vi "Sequence.Build.vi"(8 "error in (no error)":errorcluster, 11 "State Variables":T1={"Aliases.All"=[], "Aliases.Outputs"=[], "UI.Sequence#ofColumns"=0, "SysDef.Path"=path "", "UI.SequenceRef"=refnum, "UI.StepInformationRef"=refnum, "UI.AbortRef"=refnum, "UI.GraphRef"=refnum, "UI.ViewRef"=refnum, "UI.IterationsRef"=refnum, "UI.IterationInformationRef"=refnum, "INI.Settings"={"Build Location"=path "C:/Simple Sequence Editor/SequenceRepo", "LoggingLocation"=path ""}}) -> (0 "error out":errorcluster)   [LabVIEW 2013, in "Simple Sequence Tools - Editor.lvlib"]
uses:
  Simple Sequence Tools - Editor.lvlib
  Types/StateVariables.ctl
  Shared/Types/ChannelProperties.ctl
  Shared/Types/INI.Settings
  Shared/Simple Sequence Tools - Shared.lvlib
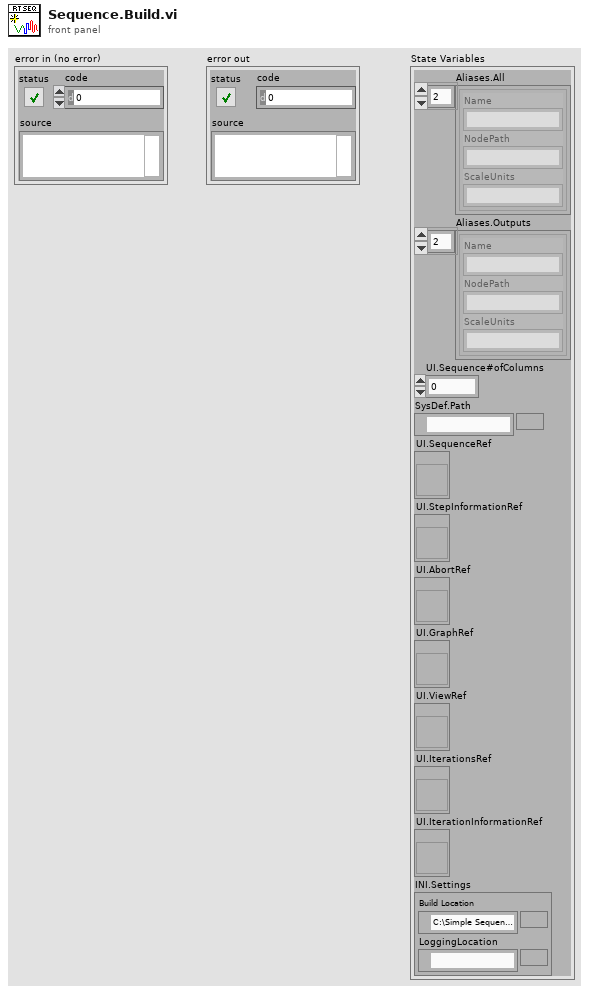
[diagram p1: front panel]
types:
  T1 = typedef "Simple Sequence Tools - Editor.lvlib/StateVariables.ctl" = cluster{"Aliases.All":T2[], "Aliases.Outputs":T2[], "UI.Sequence#ofColumns":i32, "SysDef.Path":path, "UI.SequenceRef":refnum<vi>, "UI.StepInformationRef":refnum<vi>, "UI.AbortRef":refnum<vi>, "UI.GraphRef":refnum<vi>, "UI.ViewRef":refnum<vi>, "UI.IterationsRef":refnum<vi>, "UI.IterationInformationRef":refnum<vi>, "INI.Settings":T3}
  T2 = typedef "Simple Sequence Tools - Shared.lvlib/ChannelProperties.ctl" = cluster{"Name":string, "NodePath":string, "ScaleUnits":string}
  T3 = typedef "Simple Sequence Tools - Shared.lvlib/INI.Settings" = cluster{"Build Location":path, "LoggingLocation":path}
  T4 = typedef "Simple Sequence Tools - Editor.lvlib/Compiled.RTSequenceProperties.ctl" = cluster{"Channels":T2[], "Steps":T5[], "Iterations":u32, "Sequence Channels":T11}
  T5 = typedef "Simple Sequence Tools - Editor.lvlib/Compiled.StepProperties.ctl" = cluster{"IOState":T6, "Condition":T9}
  T6 = typedef "Simple Sequence Tools - Editor.lvlib/Compiled.IOStateProperties.ctl" = cluster{"Duration":dbl, "Elements":T7[]}
  T7 = typedef "Simple Sequence Tools - Editor.lvlib/Compiled.StepElementProperties.ctl" = cluster{"Channel":T2, "Step":T8, "Parameters":dbl[]}
  T8 = typedef "Simple Sequence Tools - Shared.lvlib/StepTypes.ctl" = enum8{"Step", "iStep", "Ramp", "Unchanged", "Unknown"}
  T9 = typedef "Simple Sequence Tools - Editor.lvlib/Compiled.StepCondition.ctl" = cluster{"First Opreation":T10, "Expression":string}
  T10 = typedef "Simple Sequence Tools - Editor.lvlib/OperationTypes.ctl" = enum8{"None", "&&", "||"}
  T11 = typedef "Simple Sequence Tools - Editor.lvlib/Compiled.SequenceChannels.ctl" = cluster{"Abort":T2, "IterationInfo":T2, "StepInfo":T2}
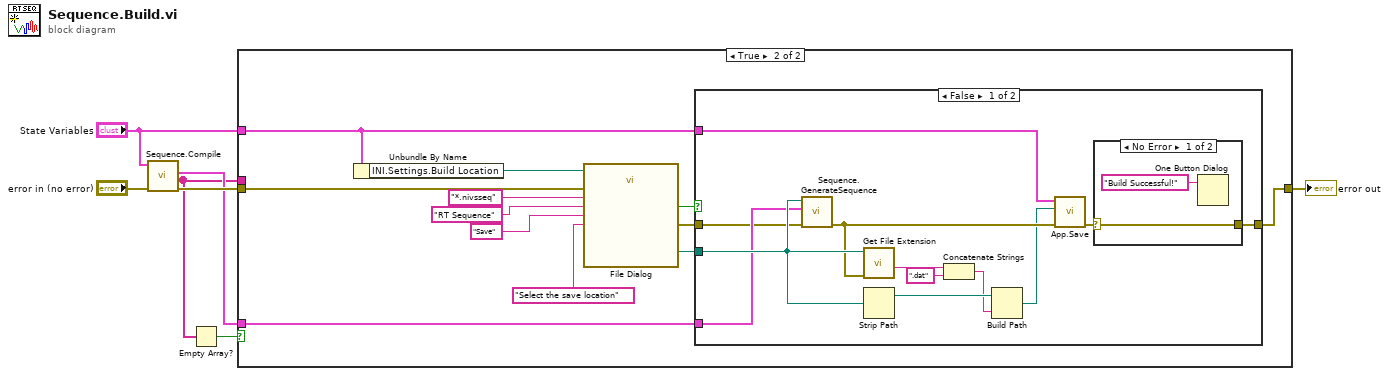
[diagram p0: block diagram]
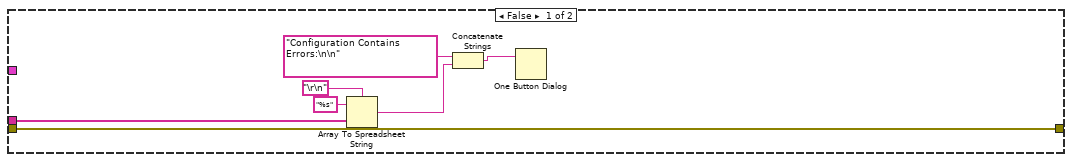
[diagram p2: hidden frame]
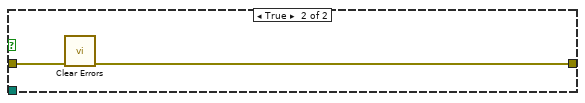
[diagram p4: hidden frame]
diagram:
  n1 = call "Sequence.Compile.vi"("error in (no error)"="error in (no error)", "State Variables"="State Variables") -> ("error out"=w5:errorcluster, "Warnings"=w1:string[], "CompiledSettings"=w4:T4)  [unwired: 7 in]
  n2 = Empty Array?(array=w1) -> (empty?=w2:bool)
  n3 = case shown="True" w2 {
    tunnel: [w14 w19] -> w7
    tunnel: w5 -> [w14 w16]
    tunnel: w4 -> [_ w18]
    tunnel: "State Variables" -> [_ w17]
    tunnel: w1 -> [w12 _]
    frame False {
      n4 = Array To Spreadsheet String(delimiter (Tab)="\r\n", array=w12, 3:"%s" ("format string")) -> (spreadsheet string=w10:string)
      n5 = Concatenate Strings("Configuration Contains Errors:\n\n", w10) -> (w13:string)
      n6 = One Button Dialog(message=w13) -> ()  [unwired: 1 in, 1 out]
    }
    frame True {
      n7 = Unbundle By Name(w17) -> ("INI.Settings.Build Location"=w15:path)
      n8 = call "File Dialog"("start path"=w15, "prompt"="Select the save location", "button label"="Save", "error in"=w16, "pattern (all files)"="*.nivsseq", "pattern label"="RT Sequence") -> ("selected path"=w24:path, "cancelled"=w25:bool, "error out"=w26:errorcluster)  [unwired: 6 in, 1 out]
      n9 = case shown="False" w25 {
        tunnel: [w27 w42] -> w19
        tunnel: w26 -> [w30 w43]
        tunnel: w24 -> [w38 _]
        tunnel: w18 -> [w31 _]
        tunnel: w17 -> [w29 _]
        frame False {
          n10 = call "Sequence.GenerateSequence.vi"("error in (no error)"=w30, "Compiled Settings"=w31, "Path"=w38) -> ("error out"=w37:errorcluster)  [unwired: 8 in]
          n11 = call <vilib>:"Get File Extension.vi"("error in (no error)"=w37, "file"=w38) -> ("filename without extension"=w35:string)  [unwired: 6 in, 3 out]
          n12 = Strip Path(path=w38) -> (stripped path=w36:path)  [unwired: 1 out]
          n13 = Concatenate Strings(w35, ".dat" ("string")) -> (w33:string)
          n14 = Build Path(base path=w36, name or relative path=w33) -> (appended path=w32:path)
          n15 = call "App.Save.vi"("error in (no error)"=w37, "selected path"=w32, "State Variables"=w29) -> ("error out"=w28:errorcluster)  [unwired: 8 in]
          n16 = case shown="No Error" w28 {
            selector: w28 -> [w40 w41]
            tunnel: [w40 w41] -> w27
            frame No Error {
              n17 = One Button Dialog(message="Build Successful!") -> ()  [unwired: 1 in, 1 out]
            }
            frame Error {
            }
          }
        }
        frame True {
          n18 = call <vilib>:"Clear Errors.vi"("error in (no error)"=w43) -> ("error out"=w42:errorcluster)  [unwired: 6 in]
        }
      }
    }
  }
  "error out" <- w7
